vi "Tenerowicz_B_2.vi"   [LabVIEW 2020]
uses:
  <vilib>/Platform/TimedLoop/XDataNode/timing_clust.ctl
  <vilib>/Platform/TimedLoop/XDataNode/nitl_modes.ctl
  <vilib>/Platform/TimedLoop/XDataNode/wakeup.ctl
  <vilib>/platform/TimedLoop/XDataNode/XDataNode.xnode
  <vilib>/Platform/TimedLoop/XDataNode/XDNodeRunTimeDep.lvlib
types:
  T1 = typedef "Rendezvous RefNum" = refnum<k1>
  T2 = typedef "Semaphore RefNum" = refnum<k1>
  T3 = typedef "XDNodeRunTimeDep.lvlib/timing_clust.ctl" = cluster{"Expected End [f-1]":u64, "Actual End [f-1]":u64, "Finished Late? [f-1]":bool, "Expected End [i-1]":u64, "Actual End [i-1]":u64, "Finished Late? [i-1]":bool, "Expected Start [i]":u64, "Actual Start [i]":u64, "Expected Start [f]":u64, "Actual Start [f]":u64, "Source Name":string, "Structure Name":string, "Period":i64, "Deadline":i64, "Offset":i64, "Start":i64, "Priority":i32, "Timeout":i32, "Mode":T4, "Wakeup Reason":T5, "Error":errorcluster, "Source Type":string, "Secondary Source Type":string, "Global End Time":u64, "Global Start Time":u64, "Frame Duration":u64, "Iteration Duration":u64, "Assigned CPU":i32, "I/O Scan Engine Mode":u32}
  T4 = typedef "XDNodeRunTimeDep.lvlib/nitl_modes.ctl" = enum32{"No Change", "Process missed periods, maintain original phase", "Discard missed periods, maintain original phase", "Process missed periods, ignore original phase", "Discard missed periods, ignore original phase"}
  T5 = typedef "XDNodeRunTimeDep.lvlib/wakeup.ctl" = enum32{"Normal", "Aborted", "Asynchronous wakeup", "Timing source error", "Timed loop error", "Timeout"}
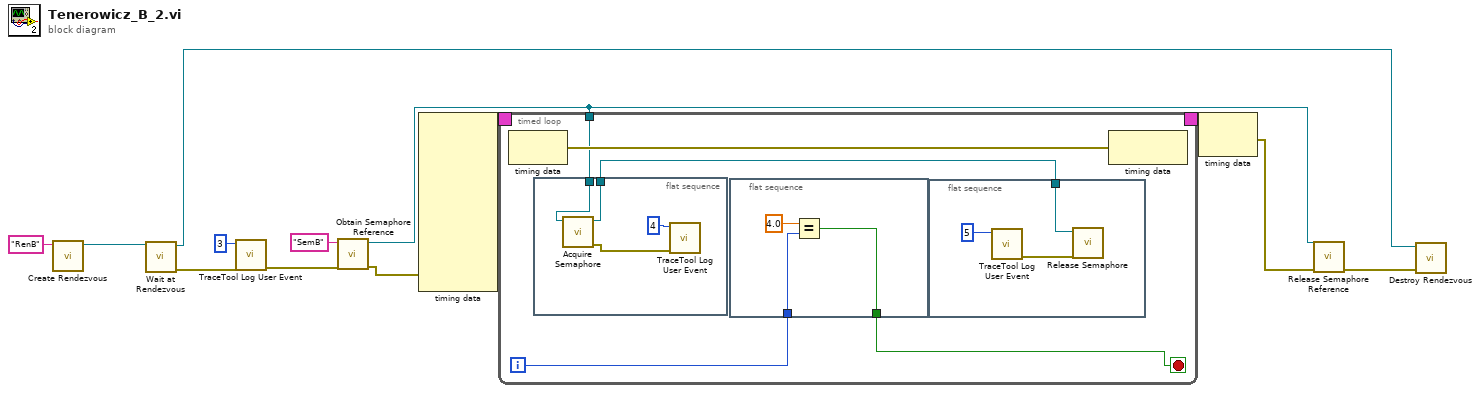
[diagram p0: block diagram]
diagram:
  n1 = call <vilib>:"Create Rendezvous.vi"("name (unnamed)"="RenB") -> ("rendezvous"=w8:T1)  [unwired: 4 in, 2 out]
  n2 = call <vilib>:"Wait at Rendezvous.vi"("rendezvous"=w8) -> ("error out"=w5:errorcluster, "rendezvous out"=w2:T1)  [unwired: 4 in, 1 out]
  n3 = call <vilib>:"TraceTool Log User Event.vi"("error in (no error)"=w5, "Event ID (0-255)"=u32 3) -> ("error out"=w4:errorcluster)  [unwired: 9 in]
  n4 = call <vilib>:"Obtain Semaphore Reference.vi"("error in (no error)"=w4, "name (unnamed)"="SemB") -> ("error out"=w3:errorcluster, "semaphore"=w1:T2)  [unwired: 3 in, 1 out]
  n5 = node-c288(w3) -> (w10:T3)  [unwired: 9 in]
  n6 = timed-loop {
    timing: w10 -> [_]
    timing-out: [_] -> w9
    tunnel: w1 -> [w15]
    i -> [w17]
    stop <- w16 stop-if-true
    n7 = node-c288() -> (w18:errorcluster)  [unwired: 1 in]
    n8 = flat-sequence {
      tunnel: w15 -> [w27]
      tunnel: [w26] -> w14
      frame #0 {
        n9 = call <vilib>:"Acquire Semaphore.vi"("semaphore"=w27) -> ("error out"=w25:errorcluster, "semaphore out"=w26:T2)  [unwired: 4 in, 1 out]
        n10 = call <vilib>:"TraceTool Log User Event.vi"("error in (no error)"=w25, "Event ID (0-255)"=u32 4) -> ()  [unwired: 9 in, 1 out]
      }
    }
    n11 = flat-sequence {
      tunnel: w17 -> [w23]
      tunnel: [w22] -> w16
      frame #0 {
        n12 = Equal?(x=4.0, y=w23) -> (x = y?=w22:bool)
      }
    }
    n13 = flat-sequence {
      tunnel: w14 -> [w20]
      frame #0 {
        n14 = call <vilib>:"TraceTool Log User Event.vi"("Event ID (0-255)"=u32 5) -> ("error out"=w19:errorcluster)  [unwired: 10 in]
        n15 = call <vilib>:"Release Semaphore.vi"("error in (no error)"=w19, "semaphore"=w20) -> ()  [unwired: 4 in, 2 out]
      }
    }
    n16 = node-c288(w18) -> ()  [unwired: 1 out]
  }
  n17 = node-c288(w9) -> (w6:errorcluster)
  n18 = call <vilib>:"Release Semaphore Reference.vi"("error in (no error)"=w6, "semaphore"=w1) -> ("error out"=w7:errorcluster)  [unwired: 8 in, 1 out]
  n19 = call <vilib>:"Destroy Rendezvous.vi"("error in (no error)"=w7, "rendezvous"=w2) -> ()  [unwired: 4 in, 2 out]
